vi "Previous Element Sum.vi"() -> ()   [LabVIEW 2025]
panel:
  out "Output Array":dbl[](array[numeric])
  in  "Input Array":dbl[](array[numeric])
  # "ME 235: Design of Microprocessor Based Mechanical Systems"
  # "Lab 2 - Previous Element Sum"
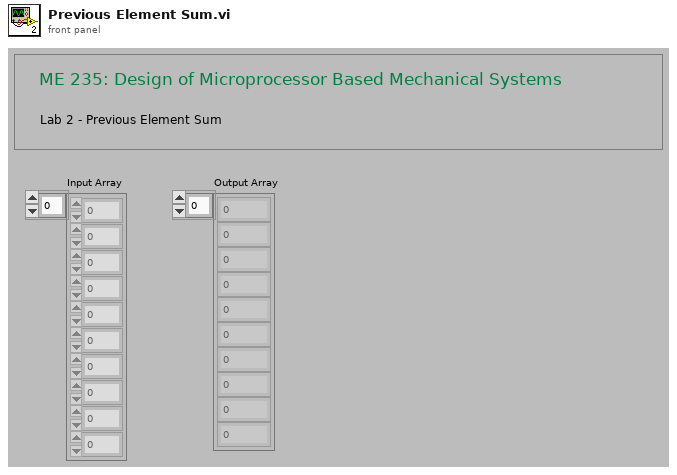
[diagram p1: front panel]
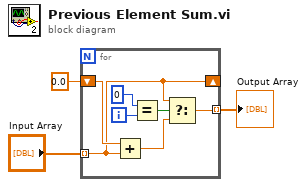
[diagram p0: block diagram]
diagram:
  n1 = for {
    tunnel: "Input Array" -> [w5] mode=indexing
    shift-right: [w5] -> _
    shift-left: 0.0 -> [w8]
    tunnel: [w4] -> w1 mode=indexing
    i -> [w9]
    n2 = Add(x=w8, y=w5) -> (x+y=w6:dbl)
    n3 = Equal?(x=0, y=w9) -> (x = y?=w7:bool)
    n4 = Select(t=w5, s=w7, f=w6) -> (s? t:f=w4:dbl)
  }
  "Output Array" <- w1
